vi "Path Manager.vi"(11 "Error in (no error)":errorcluster, 13 "Options":enum16{"Get Paths", "Init Paths"}(ring)) -> (4 "Cluster":T1, 15 "Error out":errorcluster)   [LabVIEW 2022 SP3]
uses:
  Controls/Paths.ctl
  <vilib>/Utility/sysdir.llb/System Directory Type.ctl
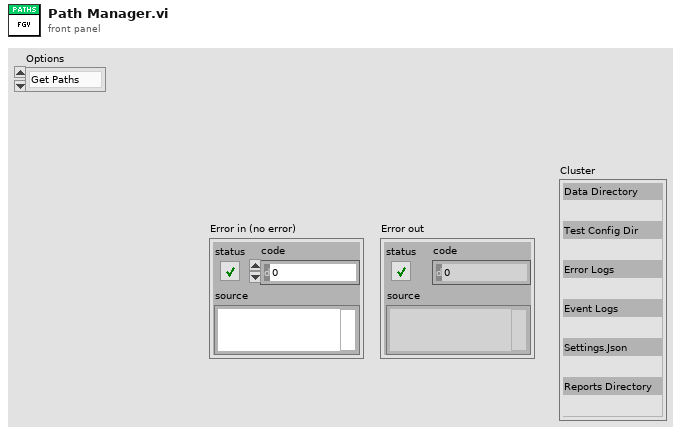
[diagram p1: front panel]
types:
  T1 = typedef "Paths.ctl" = cluster{"Data Directory":path, "Test Config Dir":path, "Error Logs":path, "Event Logs":path, "Settings.Json":path, "Reports Directory":path}
  T2 = typedef "System Directory Type.ctl" = i32
  T3 = cluster{"Array[0]":path, "Array[1]":path, "Array[2]":path, "Array[3]":path}
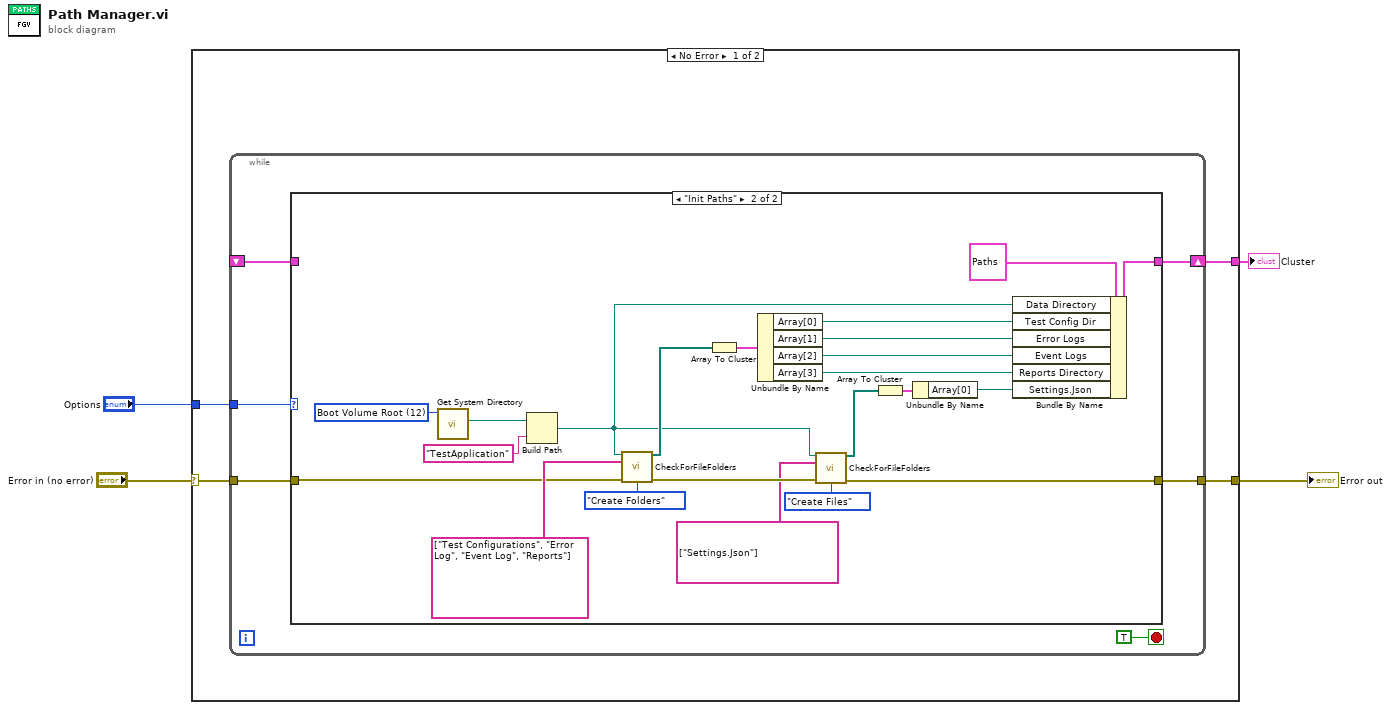
[diagram p0: block diagram]
diagram:
  n1 = case shown="No Error" "Error in (no error)" {
    selector: "Error in (no error)" -> [w8 w39]
    tunnel: [w7 w39] -> w3
    tunnel: "Options" -> [w6 _]
    tunnel: [w5 _] -> w1
    frame No Error {
      n2 = while {
        tunnel: w8 -> [w13]
        tunnel: [w12] -> w7
        tunnel: w6 -> [w14]
        shift-right: [w11] -> w5
        shift-left: _ -> [w10]
        stop <- TRUE stop-if-true
        n3 = case shown="\"Init Paths\"" w14 {
          tunnel: w13 -> [w15 w30]
          tunnel: [w15 w27] -> w12
          tunnel: [w16 w19] -> w11
          tunnel: w10 -> [w16 _]
          frame "Get Paths", Default {
          }
          frame "Init Paths" {
            w38 = T2 12 items=["User Home"=0, "User Desktop"=1, "User Documents"=2, "User Application Data"=3, "User Preferences"=4, "User Temporary"=5, "Public Documents"=6, "Public Application Data"=7, "Public Preferences"=8, "Public Cache"=13, "System Core Libraries"=9, "System Installed Libraries"=10, "Application Files"=11, "Boot Volume Root"=12] ("system directory type")
            n4 = call <vilib>:"Get System Directory.vi"("system directory type"=w38) -> ("system directory"=w37:path)  [unwired: 10 in]
            n5 = Build Path(base path=w37, name or relative path="TestApplication") -> (appended path=w18:path)
            n6 = call "CheckForFileFolders.vi"("Main Path"=w18, "Sub Path"=string[] ["Test Configurations", "Error Log", "Event Log", "Reports"], "Error in (no error)"=w30, "Operation"=enum16{"Create Files", "Create Folders"}."Create Folders") -> ("Array"=w34:path[], "Error out"=w31:errorcluster)  [unwired: 10 in]
            n7 = Array To Cluster(array=w34) -> (cluster=w32:T3)
            n8 = Unbundle By Name(w32) -> ("Array[0]"=w25:path, "Array[1]"=w24:path, "Array[2]"=w23:path, "Array[3]"=w17:path)
            n9 = call "CheckForFileFolders.vi"("Main Path"=w18, "Sub Path"=string[] ["Settings.Json"], "Error in (no error)"=w31, "Operation"=enum16{"Create Files", "Create Folders"}."Create Files") -> ("Array"=w22:path[], "Error out"=w27:errorcluster)  [unwired: 10 in]
            n10 = Array To Cluster(array=w22) -> (cluster=w21:cluster{"Array[0]":path})
            n11 = Unbundle By Name(w21) -> ("Array[0]"=w20:path)
            n12 = Bundle By Name(cluster=T1 {"Data Directory"=path "", "Test Config Dir"=path "", "Error Logs"=path "", "Event Logs"=path "", "Settings.Json"=path "", "Reports Directory"=path ""}, "Data Directory"=w18, "Test Config Dir"=w25, "Error Logs"=w24, "Event Logs"=w23, "Reports Directory"=w17, "Settings.Json"=w20) -> (w19:T1)
          }
        }
      }
    }
    frame Error {
    }
  }
  "Error out" <- w3
  "Cluster" <- w1
